vi "Config Type.vi"(11 "Digital Command in":refnum<class "Digital Command.lvclass">) -> (2 "Command Config Type":refnum<class "Command Config.lvclass">)   [LabVIEW 2020, in "VolatusSeq.lvlib" / "Digital Command.lvclass"]
uses:
  Digital Command.lvclass
  Digital Command.lvclass/Digital Command.ctl
  VolatusSeqConfig/Digital Command Config/Digital Command Config.lvclass
  C:/dev/lv20CE/relink/lv-volatus/VolatusSeqConfig/Command Config/Command Config.lvclass
  C:/dev/lv20CE/relink/lv-volatus/VolatusSeqConfig/Digital Command Config/Digital Command Config.lvclass
  VolatusSeqConfig/Command Config/Command Config.lvclass
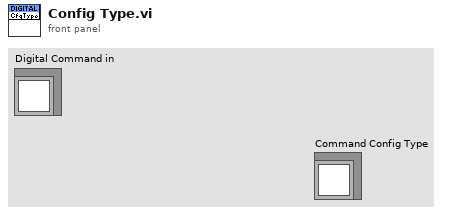
[diagram p1: front panel]
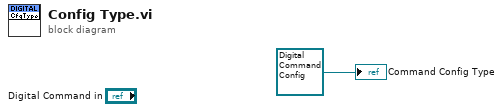
[diagram p0: block diagram]
diagram:
  "Command Config Type" <- refnum<class "Digital Command Config.lvclass"> refnum ("VolatusSeqConfig.lvlib:Digital Command Config.lvclass")
